vi "Set XY Graph Plot Colors.vi"(8 "error in (no error)":errorcluster, 10 "Colors []":u32[](array[colorbox])=[10420479, 16860, 3381759, 6618880, 16772608, 16711680], 11 "graph_utilities in":refnum<class "graph_utilities.lvclass">) -> (0 "error out":errorcluster, 3 "graph_utilities out":refnum<class "graph_utilities.lvclass">)   [LabVIEW 2016, in "graph_utilities.lvclass"]
doc: "Set the plot colors to be different according to the color table"
uses:
  graph_utilities.lvclass
  graph_utilities.lvclass/graph_utilities.ctl
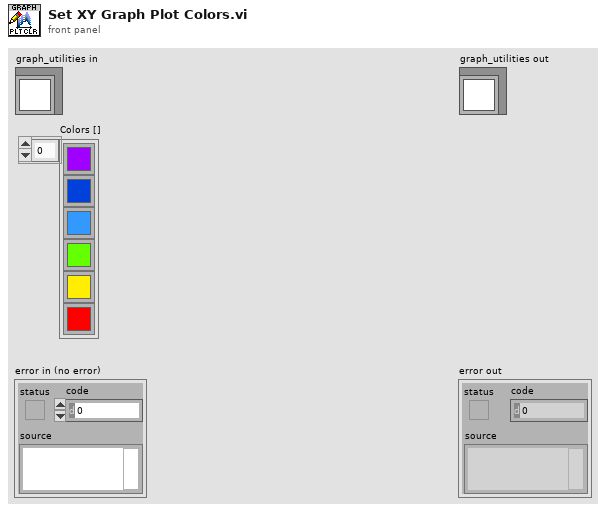
[diagram p1: front panel]
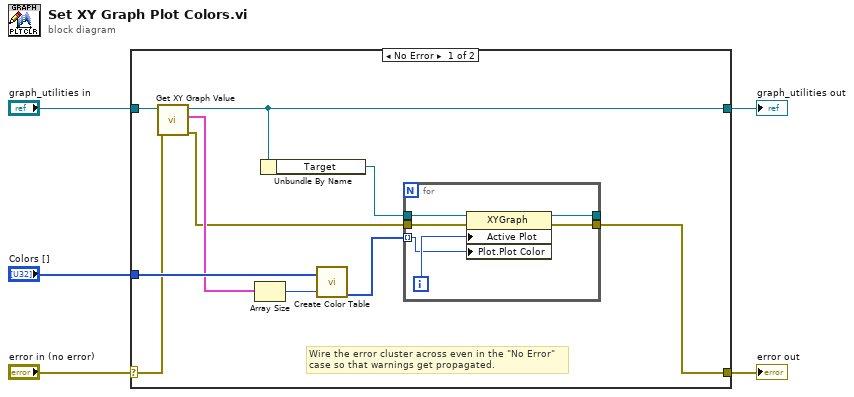
[diagram p0: block diagram]
diagram:
  n1 = case shown="No Error" "error in (no error)" {
    selector: "error in (no error)" -> [w11 w23]
    tunnel: [w15 w23] -> w4
    tunnel: [w8 w22] -> w2
    tunnel: "graph_utilities in" -> [w13 w22]
    tunnel: "Colors []" -> [w14 _]
    frame No Error {
      # "Wire the error cluster across even in the \"No Error\"\ncase so that warnings get propagated."
      n2 = call "Get XY Graph Value.vi"("error in (no error)"=w11, "graph_utilities in"=w13) -> ("error out"=w10:errorcluster, "Value"=w12:cluster{"X":dbl[], "Y":dbl[]}[], "graph_utilities out"=w8:refnum<class "graph_utilities.lvclass">)  [unwired: 7 in]
      n3 = Array Size(array=w12) -> (size(s)=w6:i32)
      n4 = Unbundle By Name(w8) -> ("Target"=w9:refnum<vi>)
      n5 = call "Create Color Table.vi"("Colors []"=w14, "Size (256)"=w6) -> ("Color Tbl"=w7:u32[])  [unwired: 3 out]
      n6 = for {
        tunnel: w7 -> [w16] mode=indexing
        tunnel: w10 -> [w21]
        tunnel: [w18] -> w15
        tunnel: w9 -> [w20]
        tunnel: [w19] -> _
        i -> [w17]
        n7 = property on="Property Node" class="XYGraph"(reference=w20, error in=w21, "Active Plot"=w17, "Plot.Plot Color"=w16) -> (reference out=w19:refnum<vi>, error out=w18:errorcluster)
      }
    }
    frame Error {
    }
  }
  "error out" <- w4
  "graph_utilities out" <- w2
